vi "PicoScopePhotoDiodeTest.vi"() -> ()   [LabVIEW 2023]
doc: "This example demonstrates how to use the PicoScope Labview library to stream data from a PicoScope 2000 Series Device"
uses:
  <instrlib>/Pico/ps2000a/PicoScope2000aLib/PicoScope2000aAnalogChannelSettings.ctl
  <instrlib>/Pico/ps2000a/PicoScope2000aLib/PicoScope2000aDigitalChannelSettings.ctl
  <vilib>/Waveform/DWDTOps.llb/DWDT Analog to Digital.vi
panel:
  in  "Standard Waveform Settings":T1={"Start Frequency"=1000.0, "Stop Frequency"=1000.0, "Increment"=0.0, "Dwell Time (seconds)"=0.0} {"Stop Frequency" min=0.03 max=1000000.0; "Start Frequency" min=0.03 max=1000000.0}
  in  "Port 0 Settings":T2={"Enabled"=FALSE, "Logic Level"=9830} {"Logic Level" items=["1.5V TTL"=9830, "2.5V CMOS"=16383]}
  in  "Channel A Settings":T3={"Enabled"=TRUE, "Coupling"=1, "Range"=6, "Analogue Offset"=0.0} {"Analogue Offset" format="%#_6p"; "Range" items=["20 mV"=1, "50 mV"=2, "100 mV"=3, "200 mV"=4, "500 mV"=5, "1 V"=6, "2 V"=7, "5 V"=8, "10 V"=9, "20 V"=10]; "Coupling" items=["AC", "DC"]}
  out "Analog Channels":T4(graph)
  out "Raw Sample Interval (sec)":dbl=1.0000000130088963e-06 format="%#.5p"
  out "Max ADC value":i16
  out "Chunk time":u32
  out "Elapsed time":dbl
  in  "Poll time (ms)":u32=10 min=1 max=1000 step=1
  in  "Data file":path=path "PicoScope2000aExampleStreaming ChA Data"
  out "size(s)":i32
  out "Queue depth":i32(graph)
  out "queue depth":i32
  in  "Buffer and Transfer Settings":T5={"startIndex"=0, "Samples"=1000000, "Down Sample Ratio"=1, "Down-Sample Mode"=0} {"Down-Sample Mode" items=["None"=0, "Aggregate"=1, "Decimate"=2, "Average"=4]; "Down Sample Ratio" step=1; "Samples" format="%_6p"}
  out "TriggeredAt (In Buffer)":u32 format="%#.6p"
  out "TriggeredAt (Total samples)":u32 format="%#.6p"
  in  "Acquisition Settings":T6={"Auto Stop"=TRUE, "Desired Sample Interval"=1, "Pre-trigger Samples"=0, "Post-trigger Samples"=1000000, "Down-Sample Ratio"=1, "Down-Sample Mode"=0, "Time Units"=3} {"Time Units" items=["Nanoseconds (ns)"=2, "Microseconds (us)"=3, "Milliseconds (ms)"=4, "Seconds (s)"=5]; "Down-Sample Mode" items=["None"=0, "Aggregate"=1, "Decimate"=2, "Average"=4]; "Post-trigger Samples" format="%#.6p"; "Pre-trigger Samples" format="%#_6p"}
  out "Port 0":digitalwaveform(graph)={"t0"=timestamp(0 s since 1904-01-01), "dt"=1.0000000130088963e-06, "Y"={"transitions"=[], "data"=[]}}
  in  "Trigger Settings":T7={"Trigger Enabled"=FALSE, "Trigger Source"=enum."Channel A", "Trigger Threshold (volts)"=0.0, "Trigger Direction"=2, "Trigger Delay (samples)"=0, "Auto Trigger Time (ms)"=1000} {"Trigger Direction" items=["Rising"=2, "Falling"=3]}
  out "Triggered":bool
  out "DownSample Interval (sec)":dbl=1.0000000130088963e-06 format="%#.5p"
  out "Total Samples":u32 format="%#.6p"
  out "Auto Stopped":bool
  in  "Serial Number":string
  in  "Open Using Serial Number":bool
  out "Number of Samples per Capture":u32 format="%#.6p"
  in  "Apply  Settings":bool
  in  "stop":bool
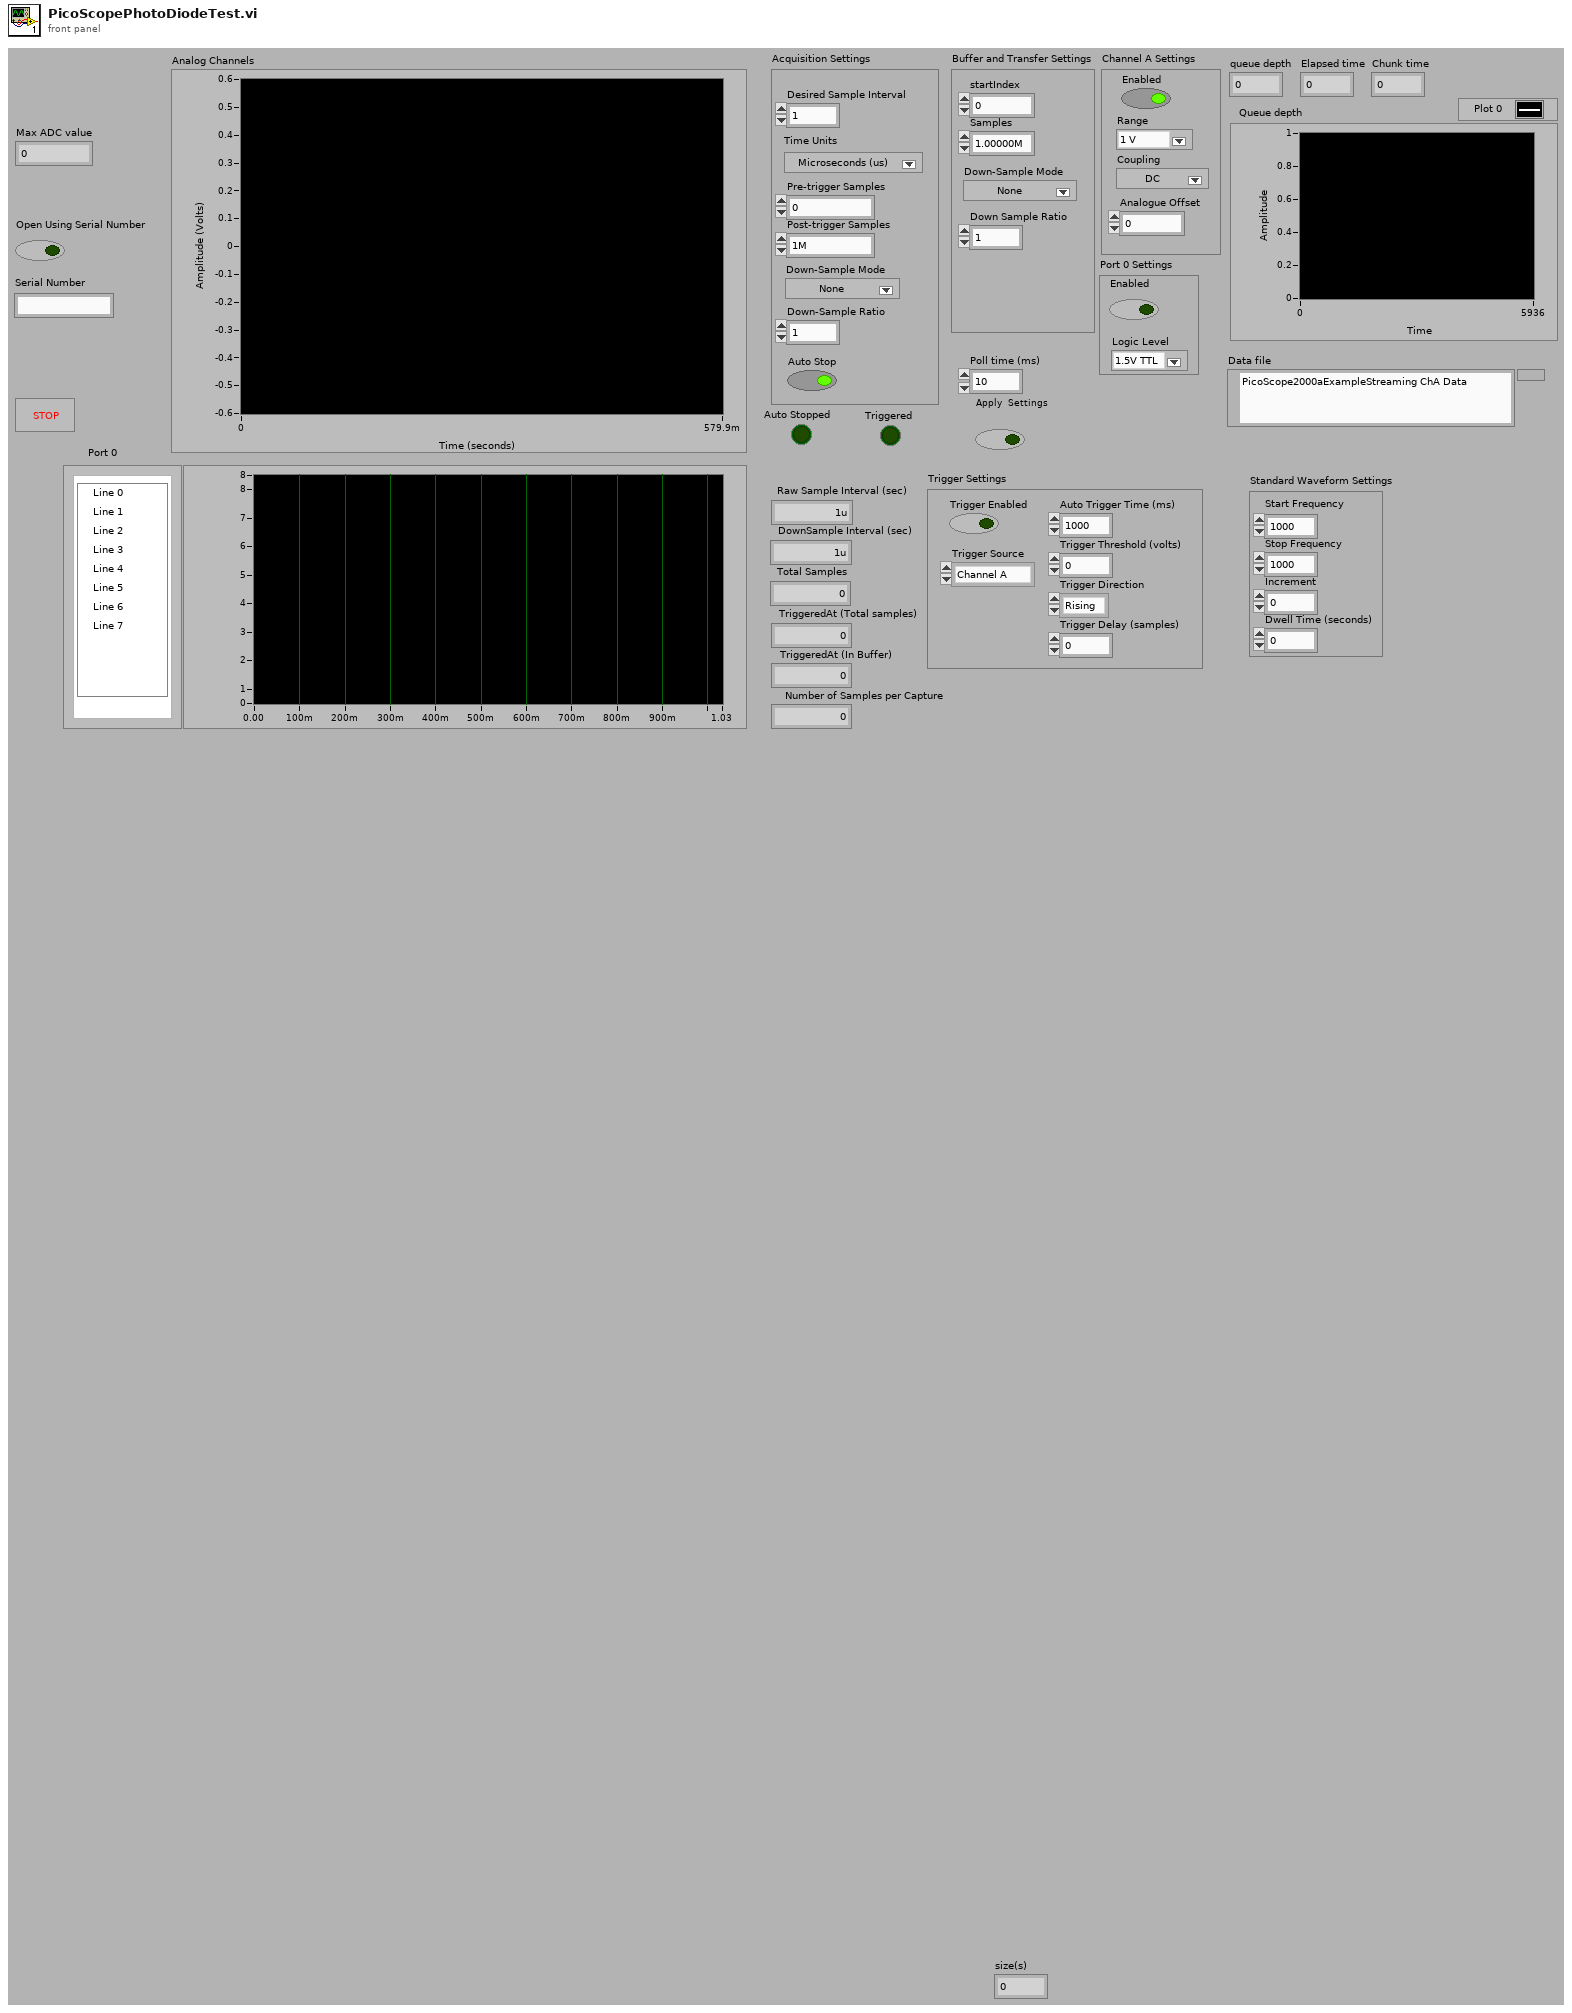
[diagram p1: front panel]
types:
  T1 = cluster{"Start Frequency":dbl, "Stop Frequency":dbl, "Increment":dbl, "Dwell Time (seconds)":dbl}
  T2 = typedef "PicoScope2000aDigitalChannelSettings.ctl" = cluster{"Enabled":bool, "Logic Level":i16}
  T3 = typedef "PicoScope2000aAnalogChannelSettings.ctl" = cluster{"Enabled":bool, "Coupling":i16, "Range":u16, "Analogue Offset":sgl}
  T4 = cluster{i32, "DownSample Interval (sec)":dbl, "Data":dbl[]}
  T5 = cluster{"startIndex":u64, "Samples":u64, "Down Sample Ratio":u64, "Down-Sample Mode":u32}
  T6 = cluster{"Auto Stop":bool, "Desired Sample Interval":u32, "Pre-trigger Samples":u32, "Post-trigger Samples":u32, "Down-Sample Ratio":u32, "Down-Sample Mode":i32, "Time Units":u32}
  T7 = cluster{"Trigger Enabled":bool, "Trigger Source":enum16{"Channel A", "Channel B", "Channel C", "Channel D", "Ext."}, "Trigger Threshold (volts)":dbl, "Trigger Direction":u16, "Trigger Delay (samples)":u32, "Auto Trigger Time (ms)":i16}
  T8 = cluster{"Peak-to-Peak Voltage (microvolts)":u32, "Offset Voltage (microvolts)":i32, "Wave Type":i16, "Sweep Type":i32, "Shots":u32, "Sweeps":u32, "Trigger Type":i32, "Trigger Source":i32, "Ext. Threshold (ADC count)":i16, "White Noise":bool}
  T9 = enum16{"open", "open or create", "create or replace", "create", "open (read-only)"}
  T10 = cluster{"Driver Version":string, "USB Version":string, "Hardware":string, "Variant":string, "Batch and Serial":string, "Cal Date":string, "Kernel Version":string, "Digital HW Version":string, "Analogue HW Version":string, "Firmware 1":string, "Firmware 2":string, "MSO":bool, "Number of Channels":i16}
  T11 = cluster{"Channel A Buffer":i16[], "Channel B Buffer":i16[], "Channel C Buffer":i16[], "Channel D Buffer":i16[], "Channel E Buffer":i16[], "Channel F Buffer":i16[], "Channel G Buffer":i16[], "Channel H Buffer":i16[], "Port 0":i16[], "Port 1":i16[]}
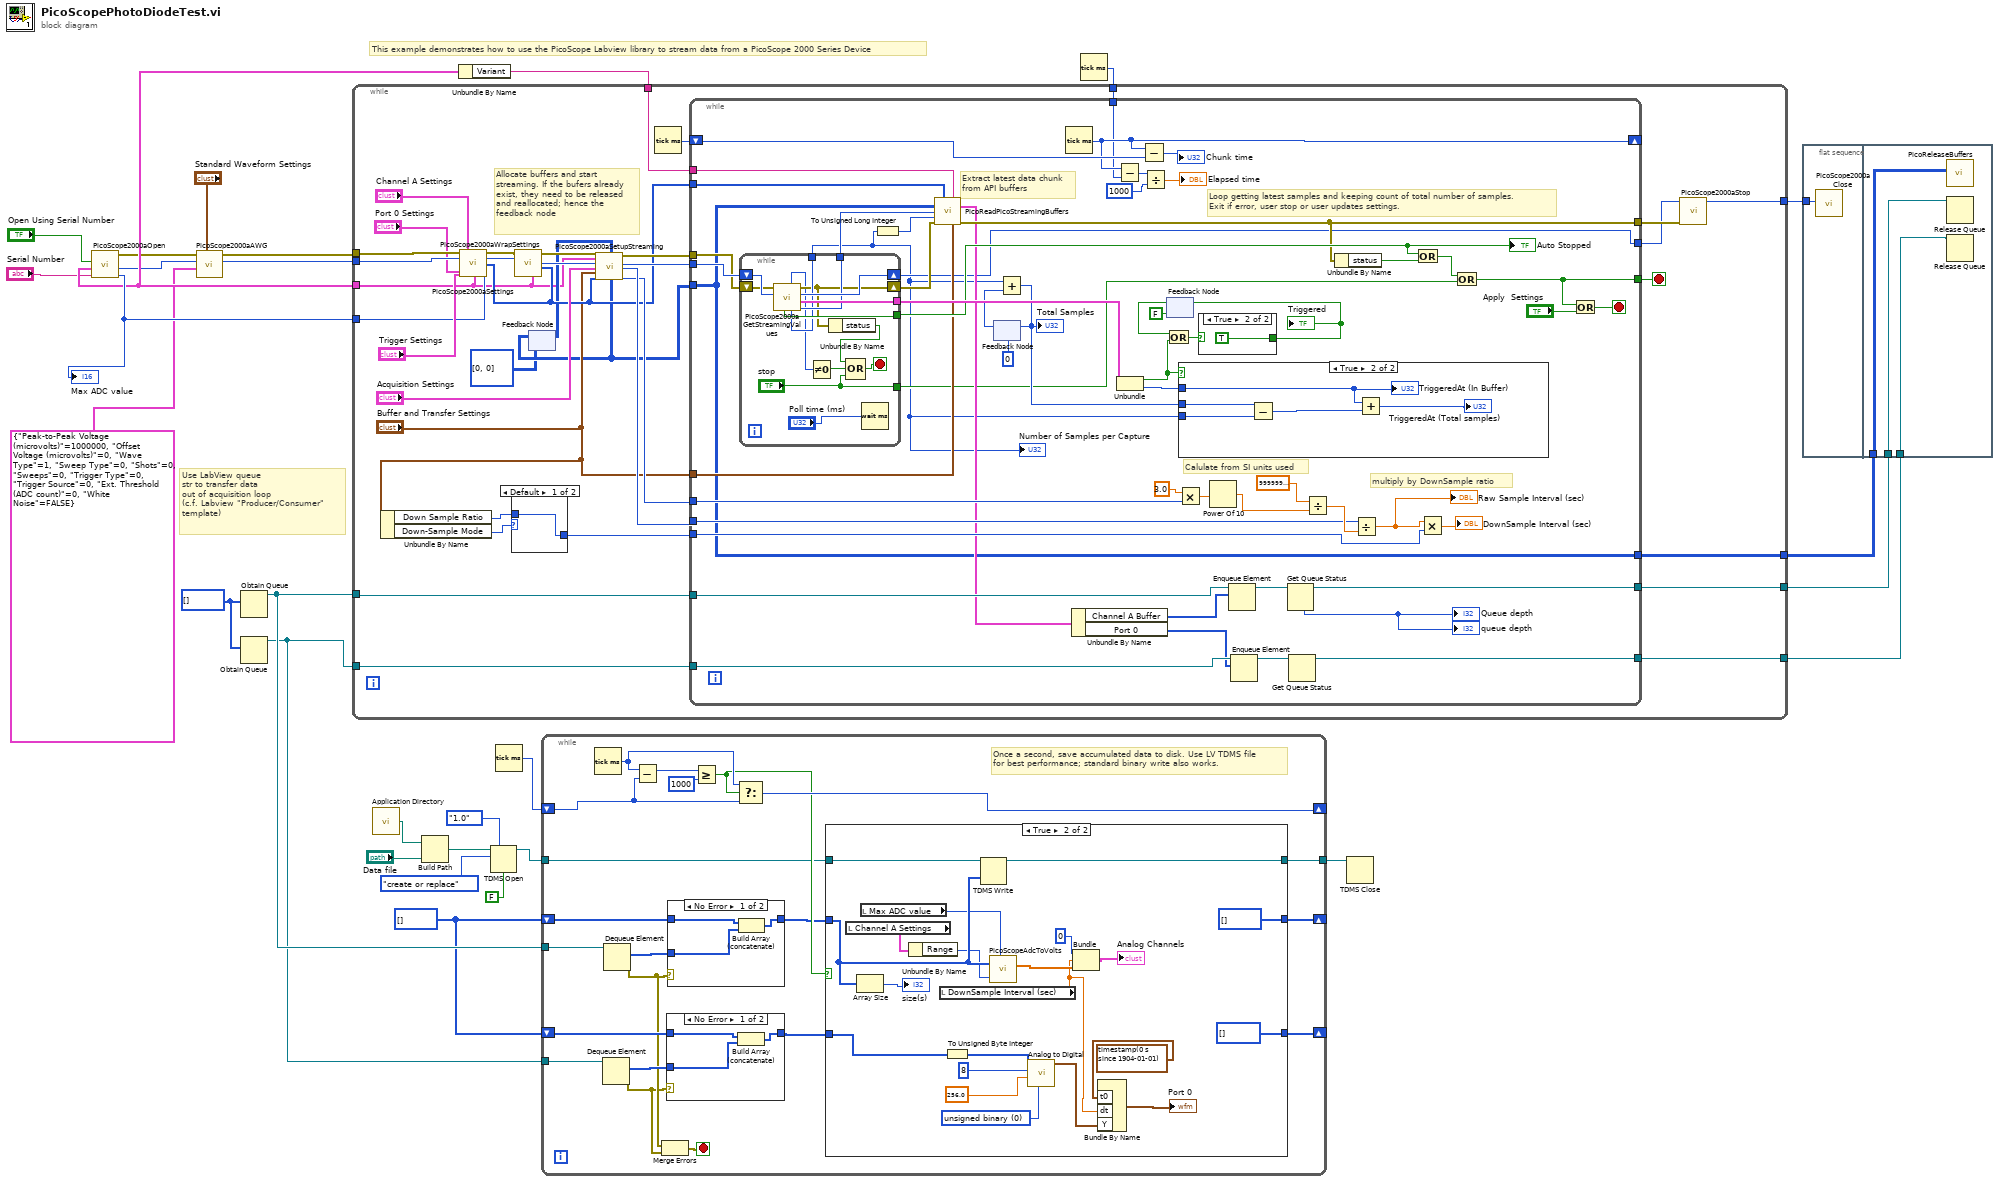
[diagram p0: block diagram]
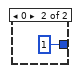
[diagram p5: hidden frame]
diagram:
  w14 = i16[] [] ("History Data")
  w17 = i16[] [] ("History Data")
  # "Use LabView queue\nstr to transfer data\nout of acquisition loop\n(c.f. Labview \"Producer/Consumer\"\ntemplate)"
  # "This example demonstrates how to use the PicoScope Labview library to stream data from a PicoScope 2000 Series Device"
  n1 = call <instrlib>:"PicoScope2000aOpen.vi"("Serial Number"="Serial Number", "Use Serial Number"="Open Using Serial Number") -> ("Max Adc value"=w29:i16, "handle"=w1:i16, "error out"=w4:errorcluster, "Device Info"=w9:T10)  [unwired: 2 in]
  "Max ADC value" <- w29
  n2 = call <instrlib>:"PicoScope2000aAWG.vi"("Standard Waveform Settings"="Standard Waveform Settings", "General AWG Settings"=T8 {"Peak-to-Peak Voltage (microvolts)"=1000000, "Offset Voltage (microvolts)"=0, "Wave Type"=1, "Sweep Type"=0, "Shots"=0, "Sweeps"=0, "Trigger Type"=0, "Trigger Source"=0, "Ext. Threshold (ADC count)"=0, "White Noise"=FALSE}, "Handle In"=w1, "error in"=w4) -> ("Handle Out"=w2:i16, "error out"=w3:errorcluster)  [unwired: 4 in, 2 out]
  n3 = Obtain Queue(element data type=w17) -> (queue out=w28:refnum<queue>)  [unwired: 4 in, 2 out]
  n4 = Obtain Queue(element data type=w17) -> (queue out=w15:refnum<queue>)  [unwired: 4 in, 2 out]
  n5 = call <vilib>:"Application Directory.vi"() -> ("Application Directory"=w11:path)
  n6 = Build Path(base path=w11, name or relative path="Data file") -> (appended path=w12:path)
  n7 = Unbundle By Name(w9) -> ("Variant"=w10:string)
  n8 = TDMS Open(6:FALSE ("disable buffering? (T)"), 7:enum16{"1.0", "2.0"}."1.0" ("file format version (2.0)"), 10:T9."create or replace" ("operation (0:open)"), 11:w12) -> (3:w21:refnum<k34>)  [unwired: 3 in, 1 out]
  n9 = Tick Count (ms)() -> (millisecond timer value=w23:u32)
  n10 = while {
    tunnel: w28 -> [w49]
    shift-right: [w40] -> _
    shift-left: w14 -> [w48]
    shift-right: [w43] -> _
    shift-left: w23 -> [w44]
    tunnel: w21 -> [w39]
    tunnel: [w38] -> w20
    tunnel: w15 -> [w36]
    shift-right: [w33] -> _
    shift-left: w14 -> [w35]
    stop <- w32 stop-if-true
    # "Once a second, save accumulated data to disk. Use LV TDMS file\nfor best performance; standard binary write also works."
    n11 = Tick Count (ms)() -> (millisecond timer value=w45:u32)
    n12 = Dequeue Element(queue=w36) -> (element=w37:i16[], error out=w30:errorcluster)  [unwired: 2 in, 2 out]
    n13 = Dequeue Element(queue=w49) -> (element=w50:i16[], error out=w31:errorcluster)  [unwired: 2 in, 2 out]
    n14 = Subtract(x=w45, y=w44) -> (x-y=w47:u32)
    n15 = Merge Errors(w31, w30) -> (w32:errorcluster)
    n16 = case shown="No Error" w30 {
      tunnel: w35 -> [w53 w54]
      tunnel: [w52 w54] -> w34
      tunnel: w37 -> [w51 _]
      frame No Error {
        n17 = Build Array (concatenate)(w53, w51) -> (w52:i16[])
      }
      frame Error {
      }
    }
    n18 = case shown="No Error" w31 {
      tunnel: w48 -> [w81 w82]
      tunnel: [w80 w82] -> w41
      tunnel: w50 -> [w79 _]
      frame No Error {
        n19 = Build Array (concatenate)(w81, w79) -> (w80:i16[])
      }
      frame Error {
      }
    }
    n20 = Greater Or Equal?(x=w47, y=u32 1000) -> (x >= y?=w42:bool)
    n21 = Select(t=w45, s=w42, f=w44) -> (s? t:f=w43:u32)
    n22 = case shown="True" w42 {
      tunnel: w41 -> [w57 w74]
      tunnel: [w57 i16[] [] ("History Data")] -> w40
      tunnel: w39 -> [w56 w76]
      tunnel: [w56 w75] -> w38
      tunnel: w34 -> [w55 w61]
      tunnel: [w55 i16[] [] ("History Data")] -> w33
      frame False {
      }
      frame True {
        w67 = u16 0 items=["unsigned binary", "offset binary", "2's complement"] ("data format (offset binary)")
        n23 = local read "Channel A Settings"() -> (w58:T3)
        n24 = Array Size(array=w74) -> (size(s)=→"size(s)":i32)
        n25 = local read "Max ADC value"() -> (w70:i16)
        n26 = Unbundle By Name(w58) -> ("Range"=w73:u16)
        n27 = local read "DownSample Interval (sec)"() -> (w62:dbl)
        n28 = To Unsigned Byte Integer(number=w61) -> (unsigned 8bit integer=w66:u8[])
        n29 = TDMS Write(0:w76, 9:w74) -> (4:w75:refnum<k34>)  [unwired: 4 in, 3 out]
        n30 = call <instrlib>:"PicoScopeAdcToVolts.vi"("Max_adc"=w70, "Range Index"=w73, "Data"=w74) -> ("Data"=w71:dbl[])
        n31 = call-poly <vilib>:"Analog to Digital.vi"("data format (offset binary)"=w67, "full-scale range (pk-pk)"=256.0, "resolution (16 bit)"=8, "analog waveform"=w66) -> ("digital waveform"=w63:digitalwaveform)  [unwired: 4 in, 3 out]
        n32 = Bundle(0, "DownSample Interval (sec)"=w62, "Data"=w71) -> (→"Analog Channels":T4)  [unwired: 1 in]
        n33 = Bundle By Name("t0"=timestamp(0 s since 1904-01-01), "dt"=w62, "Y"=w63) -> (→"Port 0":digitalwaveform)  [unwired: 1 in]
      }
    }
  }
  n34 = Tick Count (ms)() -> (millisecond timer value=w27:u32)
  n35 = while {
    tunnel: [w84] -> w26
    tunnel: w3 -> [w116]
    tunnel: w2 -> [w117]
    tunnel: w9 -> [w86]
    tunnel: w29 -> [w106]
    tunnel: [w99] -> w24
    tunnel: w28 -> [w98]
    tunnel: [w97] -> w25
    tunnel: w27 -> [w94]
    tunnel: [w91] -> w16
    tunnel: w15 -> [w90]
    tunnel: w10 -> [w89]
    stop <- w118 stop-if-true
    # "Allocate buffers and start\nstreaming. If the bufers already\nexist, they need to be released\nand reallocated; hence the\nfeedback node"
    n36 = Unbundle By Name("Buffer and Transfer Settings") -> ("Down Sample Ratio"=w103:u64, "Down-Sample Mode"=w105:u32)
    n37 = call <instrlib>:"PicoScope2000aSettings.vi"("error in"=w116, "Channel A Settings"="Channel A Settings", "handle in"=w117, "Trigger Settings"="Trigger Settings", "Port 0 Settings"="Port 0 Settings", "Device Info"=w86, "Max_adc"=w106) -> ("error out"=w111:errorcluster, "handle out"=w110:i16, "Enabled Array"=w101:i16[])  [unwired: 6 in]
    n38 = case shown="Default" w105 {
      tunnel: [w119 u32 1 ("Down-Sample Ratio")] -> w104
      tunnel: w103 -> [w119 _]
      frame Default {
      }
      frame 0 {
      }
    }
    n39 = call <instrlib>:"PicoScope2000aWrapSettings.vi"("Device Info"=w86, "Enabled array"=w101, "Handle In"=w110, "error in (no error)"=w111) -> ("Handle Out"=w113:i16, "error out"=w112:errorcluster)  [unwired: 6 in]
    n40 = feedback #1(u64[][] [[0], [0]] ("Pointer array")) -> (w96:u64[][])
    n41 = call <instrlib>:"PicoScope2000aSetupStreaming.vi"("error in"=w112, "Device Info"=w86, "handle in"=w113, "Acquisition Settings"="Acquisition Settings", "Buffer and Transfer Settings"="Buffer and Transfer Settings", "enabled array"=w101, "Pointers In"=w96) -> ("Pointer array"=w93:u64[][], "error out"=w114:errorcluster, "handle out"=w115:i16, "Sample Interval"=w108:u32, "sampleIntervalTimeUnits"=w107:u32)  [unwired: 8 in]
    n42 = feedback-in #1(w93) -> ()
    n43 = Tick Count (ms)() -> (millisecond timer value=w95:u32)
    n44 = while {
      tunnel: [w132] -> w83
      tunnel: [w175] -> w118
      tunnel: w115 -> [w151]
      tunnel: w114 -> [w150]
      tunnel: w108 -> [w154]
      tunnel: w107 -> [w162]
      tunnel: [w147] -> w85
      tunnel: w104 -> [w152]
      tunnel: "Buffer and Transfer Settings" -> [w149]
      tunnel: w101 -> [w146]
      tunnel: [w144] -> w99
      tunnel: w98 -> [w142]
      tunnel: w93 -> [w140]
      tunnel: [w140] -> w97
      shift-right: [w135] -> _
      shift-left: w95 -> [w136]
      tunnel: w94 -> [w134]
      tunnel: w89 -> [w129]
      tunnel: [w126] -> w91
      tunnel: w90 -> [w125]
      stop <- w174 stop-if-true
      # "Loop getting latest samples and keeping count of total number of samples. \nExit if error, user stop or user updates settings."
      # "Extract latest data chunk\nfrom API buffers"
      # "Calulate from SI units used"
      # "multiply by DownSample ratio"
      n45 = while {
        tunnel: [w190] -> w173
        tunnel: [w189] -> w170
        tunnel: [w185] -> w130
        tunnel: [w184] -> w121
        shift-right: [w186] -> w132
        shift-left: w151 -> [w188]
        shift-right: [w183] -> w148
        shift-left: w150 -> [w187]
        tunnel: ["stop"] -> w123
        stop <- w178 stop-if-true
        n46 = call <instrlib>:"PicoScope2000aGetStreamingValues.vi"("handle in"=w188, "error in"=w187) -> ("Start Index"=w185:u32, "Trigger"=w190:cluster{bool, "triggeredAt":u32}, "handle out"=w186:i16, "error out"=w183:errorcluster, "Number of Samples"=w184:i32, "ready"=w181:i16, "Auto Stopped"=w189:bool)  [unwired: 3 in]
        n47 = Not Equal To 0?(x=w181) -> (x != 0?=w179:bool)
        n48 = Unbundle By Name(w183) -> ("status"=w180:bool)
        n49 = Compound Arithmetic op=OR(w180, w179, "stop") -> (w178:bool)
        n50 = Wait (ms)(milliseconds to wait="Poll time (ms)") -> ()  [unwired: 1 out]
      }
      "Number of Samples per Capture" <- w121
      "Auto Stopped" <- w170
      n51 = To Unsigned Long Integer(number=w121) -> (unsigned 32bit integer=w122:u32)
      n52 = call <instrlib>:"PicoReadPicoStreamingBuffers.vi"("enabled array"=w146, "Buffer and Transfer Settings"=w149, "Variant"=w129, "Pointer array"=w140, "Offset Index"=w130, "Number of Samples"=w122, "error in (no error)"=w148) -> ("Buffers (Max or non-aggregated)"=w141:T11, "error out"=w147:errorcluster)  [unwired: 6 in, 1 out]
      n53 = feedback #2(u32 0) -> (w166:u32)
      n54 = Add(x=w121, y=w166) -> (x+y=w158:u32)
      "Total Samples" <- w158
      n55 = feedback-in #2(w158) -> ()
      n56 = Tick Count (ms)() -> (millisecond timer value=w135:u32)
      n57 = Unbundle By Name(w141) -> ("Channel A Buffer"=w131:i16[], "Port 0"=w124:i16[])
      n58 = Subtract(x=w135, y=w134) -> (x-y=w139:u32)
      n59 = Unbundle(w173) -> (w156:bool, "triggeredAt"=w155:u32)
      n60 = Subtract(x=w135, y=w136) -> (x-y=→"Chunk time":u32)
      n61 = Divide(x=w139, y=u32 1000) -> (x/y=→"Elapsed time":dbl)
      n62 = feedback #3(FALSE) -> (w168:bool)
      n63 = Or(x=w168, y=w156) -> (x .or. y?=w159:bool)
      n64 = Multiply(x=3.0, y=w162) -> (x*y=w160:dbl)
      n65 = case shown="True" w156 {
        tunnel: w121 -> [_ w191]
        tunnel: w158 -> [_ w195]
        tunnel: w155 -> [_ w193]
        frame False {
        }
        frame True {
          n66 = Subtract(x=w195, y=w191) -> (x-y=w194:u32)
          n67 = Add(x=w193, y=w194) -> (x+y=→"TriggeredAt (Total samples)":u32)
          "TriggeredAt (In Buffer)" <- w193
        }
      }
      n68 = case shown="True" w159 {
        selector: w159 -> [w196 _]
        tunnel: [w196 TRUE] -> w157
        frame False {
        }
        frame True {
        }
      }
      "Triggered" <- w157
      n69 = feedback-in #3(w157) -> ()
      n70 = Power Of 10(x=w160) -> (10^x=w161:dbl)
      n71 = Enqueue Element(queue=w142, element=w131) -> (queue out=w143:refnum<queue>)  [unwired: 2 in, 2 out]
      n72 = Enqueue Element(queue=w125, element=w124) -> (queue out=w127:refnum<queue>)  [unwired: 2 in, 2 out]
      n73 = Get Queue Status(queue=w143) -> (queue out=w144:refnum<queue>, # elements in queue=→"queue depth" →"Queue depth":i32)  [unwired: 2 in, 6 out]
      n74 = Get Queue Status(queue=w127) -> (queue out=w126:refnum<queue>)  [unwired: 2 in, 7 out]
      n75 = Divide(x=sgl 1000000000000000.0 ("y"), y=w161) -> (x/y=w163:dbl)
      n76 = Unbundle By Name(w147) -> ("status"=w172:bool)
      n77 = Divide(x=w154, y=w163) -> (x/y=w128:dbl)
      "Raw Sample Interval (sec)" <- w128
      n78 = Or(x=w170, y=w172) -> (x .or. y?=w171:bool)
      n79 = Multiply(x=w128, y=w152) -> (x*y=→"DownSample Interval (sec)":dbl)
      n80 = Or(x=w171, y=w123) -> (x .or. y?=w175:bool)
      n81 = Or(x=w175, y="Apply  Settings") -> (x .or. y?=w174:bool)
    }
    n82 = call <instrlib>:"PicoScope2000aStop.vi"("error in (no error)"=w85, "handle in"=w83) -> ("handle out"=w84:i16)  [unwired: 8 in, 1 out]
  }
  n83 = TDMS Close(11:w20) -> ()  [unwired: 1 in, 2 out]
  n84 = flat-sequence {
    tunnel: w26 -> [w198]
    tunnel: w25 -> [w201]
    tunnel: w24 -> [w200]
    tunnel: w16 -> [w199]
    frame #0 {
      n85 = call <instrlib>:"PicoScope2000aClose.vi"("handle"=w198) -> ()
    }
    frame #1 {
      n86 = call <instrlib>:"PicoReleaseBuffers.vi"("Pointer array"=w201) -> ()  [unwired: 10 in, 1 out]
      n87 = Release Queue(queue=w200) -> ()  [unwired: 2 in, 3 out]
      n88 = Release Queue(queue=w199) -> ()  [unwired: 2 in, 3 out]
    }
  }
